vi "3.11-Convert X Y to Critical Points.vi"(1 "Y (mm)":dbl[](array[numeric])=[-824.0, -821.8748054185536, -817.5016965016204, -818.8762184987505, -802.0414964088986, -800.9405372657634, -800.59012577146, -788.0816444032098, -786.2728465808068, -784.2245424325394, -781.9373558916932, -787.2650011250265, -784.474375788512, -778.521681763403, -776.2365810207972, -783.3658451204344, 730.5588889131224, 725.4102955430903, 724.8109075281693, 724.931328200215, 718.9384865393471, 714.6245895498994, 721.8640829579484, 720.0248002938554, 725.866494387571, 726.5437830014478, 731.9681149910491, 736.1878818898, 736.2022690917503, 745.9762624616667, 740.54860282115, 736.8877513302604, 737.0, -580.0, -600.0, -620.0, -640.0, -660.0, -680.0, -700.0, -720.0, -740.0, -760.0, -780.0, -800.0, -820.0, -840.0, -860.0, -880.0, -900.0, -920.0, -940.0, -960.0, -980.0, -1000.0, -1020.0, -1040.0, -1060.0, -1080.0, -1100.0, -1120.0, -1140.0, -1160.0, 580.0, 600.0, 620.0, 640.0, 660.0, 680.0, 700.0, 720.0, 740.0, 760.0, 780.0, 800.0, 820.0, 840.0, 860.0, 880.0, 900.0, 920.0, 940.0, 960.0, 980.0, 1000.0, 1020.0, 1040.0, 1060.0, 1080.0, 1100.0, 1120.0, 1140.0, 1160.0], 2 "X (mm)":dbl[](array[numeric])=[840.0, 854.3458780914469, 868.5477883026458, 882.9154841192139, 896.0842048902769, 910.0732171691171, 924.145412930461, 936.7642586636871, 950.5034421622921, 964.2089652419434, 977.8766530675427, 993.028814291989, 1006.7451760358431, 1019.7358924207481, 1033.5375164797342, 1049.9022455781442, 1049.4843904209192, 1034.373102871993, 1020.7156560129519, 1007.3635844318354, 992.8150927510532, 978.9089486341247, 967.2841142298599, 954.0407250143282, 942.0138830037281, 929.2083593725679, 916.9329489649929, 904.4080938905194, 891.4802776231645, 879.0949593134791, 865.8605270565532, 852.8624235442778, 840.0, 0.0, 0.0, 0.0, 0.0, 0.0, 0.0, 0.0, 0.0, 0.0, 0.0, 0.0, 0.0, 0.0, 0.0, 0.0, 0.0, 0.0, 0.0, 0.0, 0.0, 0.0, 0.0, 0.0, 0.0, 0.0, 0.0, 0.0, 0.0, 0.0, 0.0, 0.0, 0.0, 0.0, 0.0, 0.0, 0.0, 0.0, 0.0, 0.0, 0.0, 0.0, 0.0, 0.0, 0.0, 0.0, 0.0, 0.0, 0.0, 0.0, 0.0, 0.0, 0.0, 0.0, 0.0, 0.0, 0.0, 0.0, 0.0, 0.0, 0.0]) -> (0 "Array":T1(array[cluster]))   [LabVIEW 2010]
uses:
  3.0-Global.vi
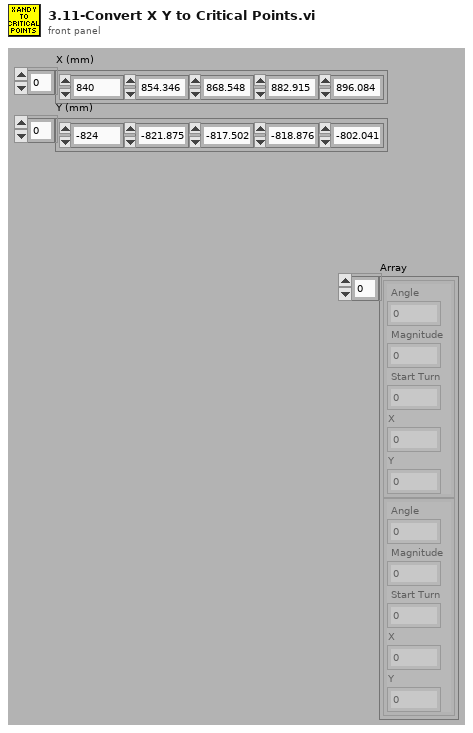
[diagram p1: front panel]
types:
  T1 = cluster{" Angle":dbl, " Magnitude":dbl, " Start Turn":dbl, "X":dbl, "Y":dbl}[]
  T2 = cluster{"Right Angle":dbl, "Right Magnitude":dbl, "Right Start Turn":dbl, "X":dbl, "Y":dbl}
  T3 = cluster{"Left Angle":dbl, "Left Magnitude":dbl, "Left Start Turn":dbl, "X":dbl, "Y":dbl}
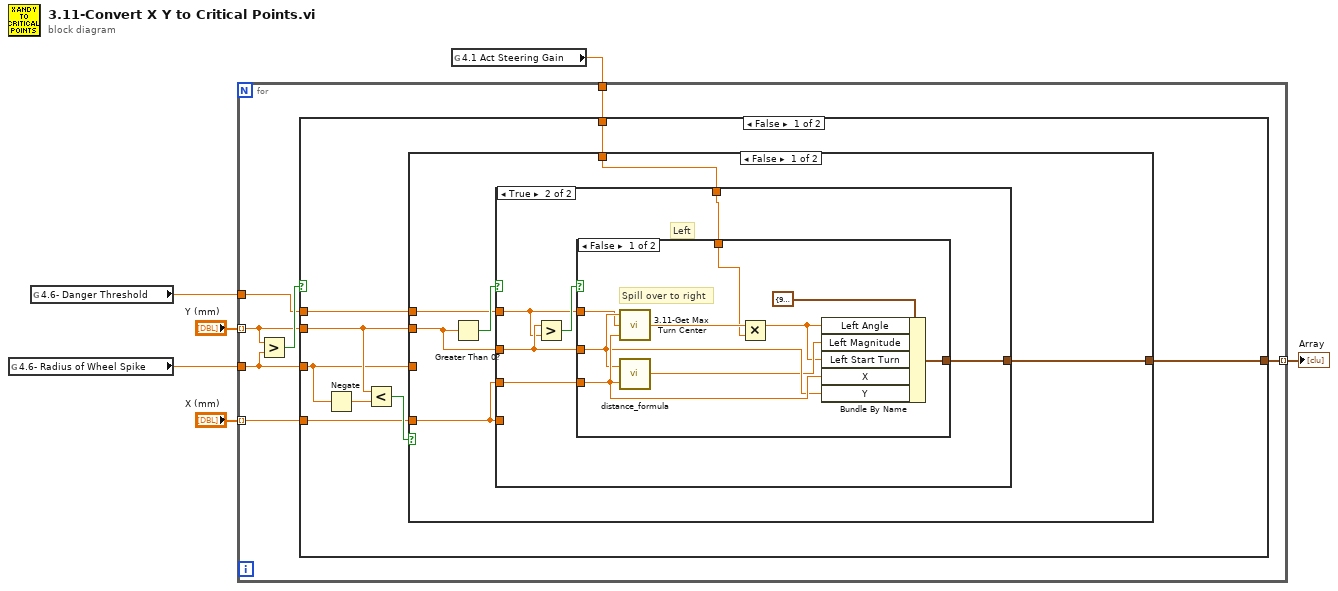
[diagram p0: block diagram]
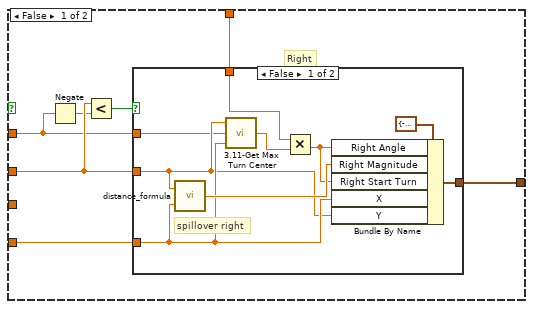
[diagram p2: hidden frame]
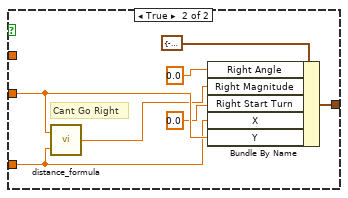
[diagram p3: hidden frame]
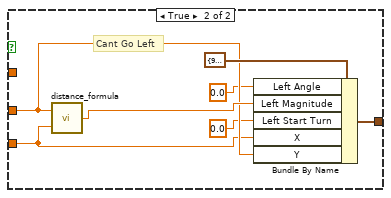
[diagram p4: hidden frame]
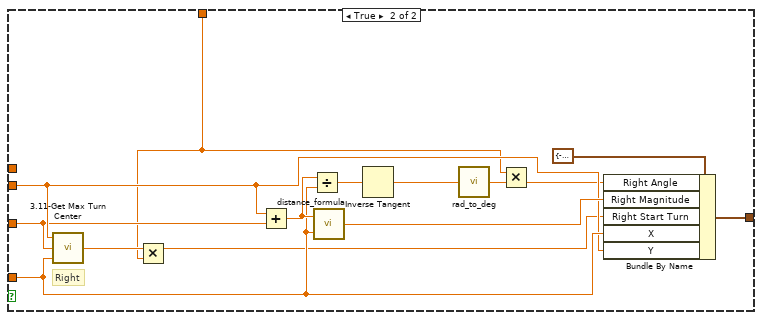
[diagram p5: hidden frame]
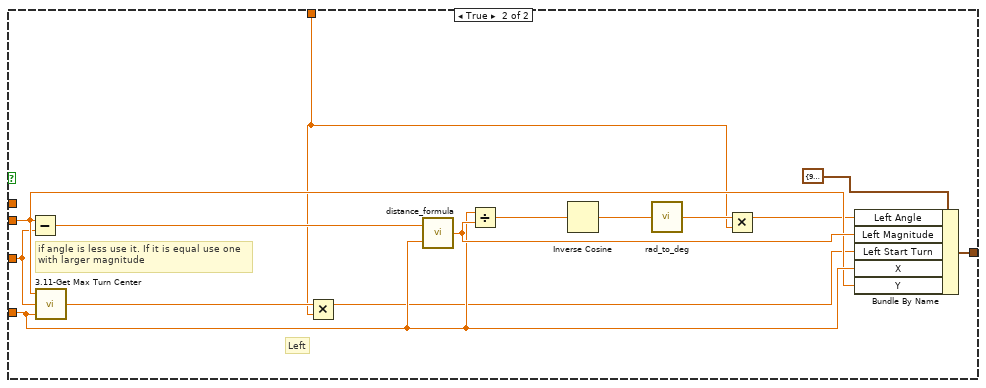
[diagram p6: hidden frame]
diagram:
  n1 = global read "3.0-Global.vi" "4.6- Radius of Wheel Spike"() -> (w3:dbl)
  n2 = global read "3.0-Global.vi" "4.6- Danger Threshold"() -> (w2:dbl)
  n3 = global read "3.0-Global.vi" "4.1 Act Steering Gain"() -> (w1:dbl)
  n4 = for {
    tunnel: "Y (mm)" -> [w12] mode=indexing
    tunnel: "X (mm)" -> [w11] mode=indexing
    tunnel: [w10] -> w6 mode=indexing
    tunnel: w3 -> [w9]
    tunnel: w2 -> [w8]
    tunnel: w1 -> [w7]
    n5 = Greater?(x=w12, y=w9) -> (0:w13:bool)
    n6 = case shown="False" w13 {
      tunnel: w12 -> [w19 w93]
      tunnel: w11 -> [w20 w94]
      tunnel: [w18 w91] -> w10
      tunnel: w9 -> [w16 w90]
      tunnel: w8 -> [w15 _]
      tunnel: w7 -> [w14 w87]
      frame False {
        n7 = Negate(x=w16) -> (-x=w17:dbl)
        n8 = Less?(x=w19, y=w17) -> (x < y?=w21:bool)
        n9 = case shown="False" w21 {
          tunnel: w20 -> [w25 w79]
          tunnel: w19 -> [w26 w78]
          tunnel: [w24 w77] -> w18
          tunnel: w16 -> [_ w76]
          tunnel: w15 -> [w23 _]
          tunnel: w14 -> [w22 w73]
          frame False {
            n10 = Greater Than 0?(x=w26) -> (x > 0?=w27:bool)
            n11 = case shown="True" w27 {
              tunnel: w26 -> [w33 w55]
              tunnel: w25 -> [_ w54]
              tunnel: w25 -> [w32 _]
              tunnel: [w31 w53] -> w24
              tunnel: w23 -> [w29 w52]
              tunnel: w22 -> [w28 w51]
              frame False {
                # "Right"
                n12 = Negate(x=w29) -> (-x=w30:dbl)
                n13 = Less?(x=w33, y=w30) -> (x < y?=w34:bool)
                n14 = case shown="False" w34 {
                  tunnel: w33 -> [w38 w49]
                  tunnel: w32 -> [w39 w48]
                  tunnel: [w42 w44] -> w31
                  tunnel: w29 -> [w37 _]
                  tunnel: w28 -> [w35 _]
                  frame False {
                    # "spillover right"
                    n15 = call "distance_formula.vi"("X2 - X1"=w39, "Y2 - Y1"=w38) -> ("Distance"=w40:dbl)
                    n16 = call "3.11-Get Max Turn Center.vi"("X (mm)"=w39, "Distance Along Y where polar system is centered"=w37, "Y (mm)"=w38) -> ("Start Turn Angle"=w41:dbl)
                    n17 = Multiply(x=w35, y=w41) -> (x*y=w36:dbl)
                    n18 = Bundle By Name(cluster=T2 {"Right Angle"=-90.0, "Right Magnitude"=0.0, "Right Start Turn"=-90.0, "X"=-1.0, "Y"=-1701.0} ("input cluster"), "Right Angle"=w36, "Right Magnitude"=w40, "Right Start Turn"=w36, "X"=w39, "Y"=w38) -> (w42:T2)
                  }
                  frame True {
                    # "Cant Go Right"
                    n19 = call "distance_formula.vi"("X2 - X1"=w48, "Y2 - Y1"=w49) -> ("Distance"=w47:dbl)
                    n20 = Bundle By Name(cluster=T2 {"Right Angle"=-90.0, "Right Magnitude"=0.0, "Right Start Turn"=-90.0, "X"=-1.0, "Y"=-1701.0} ("input cluster"), "Right Angle"=0.0 ("y"), "Right Magnitude"=w47, "Right Start Turn"=0.0 ("y"), "X"=w48, "Y"=w49) -> (w44:T2)
                  }
                }
              }
              frame True {
                # "Left"
                n21 = Greater?(x=w55, y=w52) -> (0:w56:bool)
                n22 = case shown="False" w56 {
                  tunnel: w55 -> [w63 w70]
                  tunnel: w54 -> [w64 w69]
                  tunnel: [w60 w66] -> w53
                  tunnel: w52 -> [w59 _]
                  tunnel: w51 -> [w57 _]
                  frame False {
                    # "Spill over to right"
                    n23 = call "3.11-Get Max Turn Center.vi"("X (mm)"=w64, "Distance Along Y where polar system is centered"=w59, "Y (mm)"=w63) -> ("Start Turn Angle"=w62:dbl)
                    n24 = call "distance_formula.vi"("X2 - X1"=w64, "Y2 - Y1"=w63) -> ("Distance"=w61:dbl)
                    n25 = Multiply(x=w62, y=w57) -> (x*y=w58:dbl)
                    n26 = Bundle By Name(cluster=T3 {"Left Angle"=90.0, "Left Magnitude"=0.0, "Left Start Turn"=90.0, "X"=-1.0, "Y"=1701.0} ("input cluster"), "Left Angle"=w58, "Left Magnitude"=w61, "Left Start Turn"=w58, "X"=w64, "Y"=w63) -> (w60:T3)
                  }
                  frame True {
                    # "Cant Go Left"
                    n27 = call "distance_formula.vi"("X2 - X1"=w69, "Y2 - Y1"=w70) -> ("Distance"=w71:dbl)
                    n28 = Bundle By Name(cluster=T3 {"Left Angle"=90.0, "Left Magnitude"=0.0, "Left Start Turn"=90.0, "X"=-1.0, "Y"=1701.0} ("input cluster"), "Left Angle"=0.0 ("y"), "Left Magnitude"=w71, "Left Start Turn"=0.0 ("y"), "X"=w69, "Y"=w70) -> (w66:T3)
                  }
                }
              }
            }
          }
          frame True {
            # "Right"
            n29 = call "3.11-Get Max Turn Center.vi"("X (mm)"=w79, "Distance Along Y where polar system is centered"=w76, "Y (mm)"=w78) -> ("Start Turn Angle"=w81:dbl)
            n30 = Multiply(x=w81, y=w73) -> (x*y=w75:dbl)
            n31 = Add(x=w78, y=w76) -> (x+y=w85:dbl)
            n32 = Divide(x=w85, y=w79) -> (x/y=w86:dbl)
            n33 = call "distance_formula.vi"("X2 - X1"=w79, "Y2 - Y1"=w85) -> ("Distance"=w80:dbl)
            n34 = Inverse Tangent(1:w86) -> (0:w82:dbl)
            n35 = call "rad_to_deg.vi"("Radians"=w82) -> ("Degrees"=w83:dbl)
            n36 = Multiply(x=w73, y=w83) -> (x*y=w74:dbl)
            n37 = Bundle By Name(cluster=T2 {"Right Angle"=-90.0, "Right Magnitude"=0.0, "Right Start Turn"=-90.0, "X"=-1.0, "Y"=-1701.0} ("input cluster"), "Right Angle"=w74, "Right Magnitude"=w80, "Right Start Turn"=w75, "X"=w79, "Y"=w78) -> (w77:T2)
          }
        }
      }
      frame True {
        # "if angle is less use it. If it is equal use one\nwith larger magnitude"
        # "Left"
        n38 = Subtract(x=w93, y=w90) -> (x-y=w100:dbl)
        n39 = call "3.11-Get Max Turn Center.vi"("X (mm)"=w94, "Distance Along Y where polar system is centered"=w90, "Y (mm)"=w93) -> ("Start Turn Angle"=w92:dbl)
        n40 = Multiply(x=w92, y=w87) -> (x*y=w88:dbl)
        n41 = call "distance_formula.vi"("X2 - X1"=w94, "Y2 - Y1"=w100) -> ("Distance"=w95:dbl)
        n42 = Divide(x=w94, y=w95) -> (x/y=w99:dbl)
        n43 = Inverse Cosine(1:w99) -> (0:w97:dbl)
        n44 = call "rad_to_deg.vi"("Radians"=w97) -> ("Degrees"=w96:dbl)
        n45 = Multiply(x=w96, y=w87) -> (x*y=w89:dbl)
        n46 = Bundle By Name(cluster=T3 {"Left Angle"=90.0, "Left Magnitude"=0.0, "Left Start Turn"=90.0, "X"=-1.0, "Y"=1701.0} ("input cluster"), "Left Angle"=w89, "Left Magnitude"=w95, "Left Start Turn"=w88, "X"=w94, "Y"=w93) -> (w91:T3)
      }
    }
  }
  "Array" <- w6
